vi "FestoCPX.DI.Read.vi"(8 "error in (no error)":errorcluster, 11 "TCP Conn Ref":refnum<k5>) -> (0 "error out":errorcluster, 3 "TCP Conn Ref out":refnum<k5>)   [LabVIEW 2016]
uses:
  FestoCPX.DI.Data.Fglb.Action.ctl
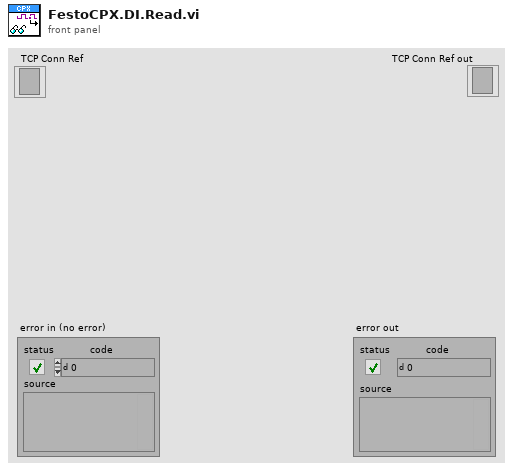
[diagram p1: front panel]
types:
  T1 = typedef "FestoCPX.DI.Data.Fglb.Action.ctl" = enum16{"init", "set", "simul", "get"}
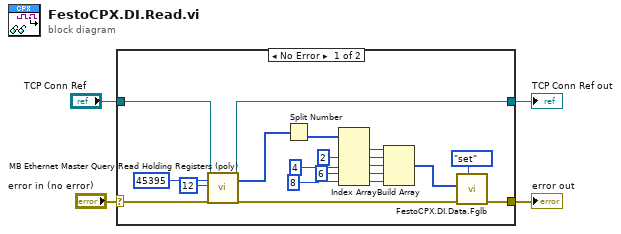
[diagram p0: block diagram]
diagram:
  n1 = case shown="No Error" "error in (no error)" {
    selector: "error in (no error)" -> [w10 w25]
    tunnel: "TCP Conn Ref" -> [w9 w26]
    tunnel: [w11 w26] -> w3
    tunnel: [w6 w25] -> w1
    frame No Error {
      n2 = call "MB Ethernet Master Query Read Holding Registers (poly).vi"("TCP Connection Refnum in"=w9, "Starting Address"=u16 45395, "Quantity"=u16 12, "error in"=w10) -> ("TCP Connection Refnum (dup)"=w11:refnum<k5>, "Holding Registers"=w22:u16[], "error out"=w7:errorcluster)  [unwired: 12 in, 1 out]
      n3 = Split Number(x=w22) -> (lo(x)=w14:u8[])  [unwired: 1 out]
      n4 = Index Array(array=w14, index #2=2 ("index"), index #3=4 ("index"), index #4=6 ("index"), index #5=8 ("index")) -> (element #1=w17:u8, element #2=w16:u8, element #3=w15:u8, element #4=w13:u8, element #5=w12:u8)  [unwired: 1 in]
      n5 = Build Array(w17, w16, w15, w13, w12) -> (w5:u8[])
      n6 = call "FestoCPX.DI.Data.Fglb.vi"("state (get)"=FestoCPX.DI.Data.Fglb.Action."set", "error in (no error)"=w7, "data bytes"=w5) -> ("error out"=w6:errorcluster)  [unwired: 4 in, 4 out]
    }
    frame Error {
    }
  }
  "error out" <- w1
  "TCP Conn Ref out" <- w3
